vi "CalculateFilterRange.vi"(6 "n":i32=84, 9 "df":dbl=0.732421875, 10 "f_0":dbl=199.951171875, 11 "Semitone":dbl=0.5) -> (2 "range":i32=21, 3 "start":i32=74)   [LabVIEW 2022 SP3]
panel:
  out "Low":dbl=254.0
  out "High":dbl=269.0
  out "frequency":dbl=261.474609375
  # "G3\t196.00\t176.02\n G#3/Ab3 \t207.65\t166.14\nA3\t220.00\t156.82\n A#3/Bb3 \t233.08\t148.02\nB3\t246.94\t139.71\nC4\t261.63\t131.87\n C#4/Db4 \t277.18\t124.47\nD4\t293.66\t117.48\n D#4/Eb4 \t311.13\t110.89\nE4\t329.63\t104.66\nF4\t349.23\t98.79\n F#4/Gb4 \t369.99\t93.24\nG4\t392.00\t88.01\n G#4/Ab4 \t415.30\t83.07\nA4\t440.00\t78.41\n A#4/Bb4 \t466.16\t74.01\nB4\t493.88\t69.85\nC5\t523.25\t65.93\n C#5/Db5 \t554.37\t62.23\nD5\t587.33\t58.74\n D#5/Eb5 \t622.25\t55.44"
  # "84 is close to C4\n587 is close to D5"
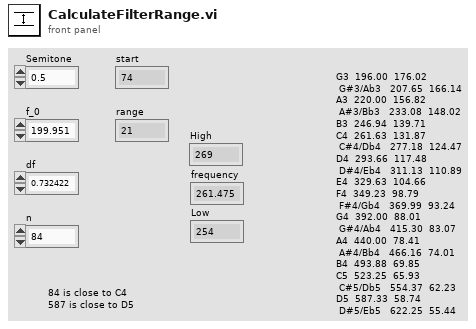
[diagram p1: front panel]
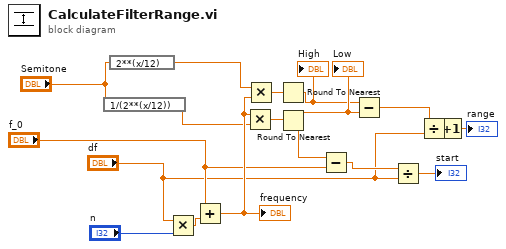
[diagram p0: block diagram]
diagram:
  n1 = expression code="1/(2**(x/12))"("Semitone") -> (w8:dbl)
  n2 = expression code="2**(x/12)"("Semitone") -> (w7:dbl)
  n3 = Multiply(x="df", y="n") -> (x*y=w13:dbl)
  n4 = Add(x="f_0", y=w13) -> (x+y=w14:dbl)
  "frequency" <- w14
  n5 = Multiply(x=w14, y=w8) -> (x*y=w10:dbl)
  n6 = Multiply(x=w7, y=w14) -> (x*y=w9:dbl)
  n7 = Round To Nearest(number=w9) -> (nearest integer value=w11:dbl)
  "High" <- w11
  n8 = Round To Nearest(number=w10) -> (nearest integer value=w16:dbl)
  "Low" <- w16
  n9 = Subtract(x=w16, y="f_0") -> (x-y=w15:dbl)
  n10 = Subtract(x=w11, y=w16) -> (x-y=w2:dbl)
  n11 = Divide(x=w15, y="df") -> (x/y=→"start":dbl)
  n12 = Divide(x=w2, y="df") -> (x/y=w3:dbl)
  n13 = Increment(x=w3) -> (x+1=→"range":dbl)
